vi "PRACTICA 1 REV.vi"() -> ()   [LabVIEW 2017]
panel:
  in  "stop":bool
  out "X+Y 2":dbl
  out "X+Y":dbl
  in  "Y":dbl
  in  "X":dbl
  out "C":dbl
  in  "B":dbl
  in  "A":dbl
  out "Boolean":bool
  # "-"
  # "="
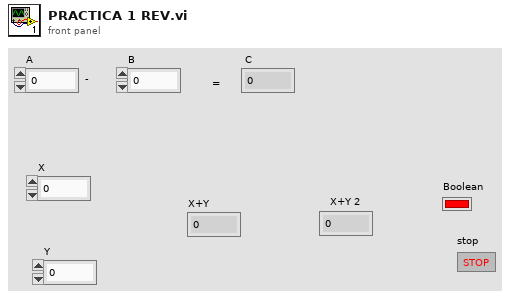
[diagram p1: front panel]
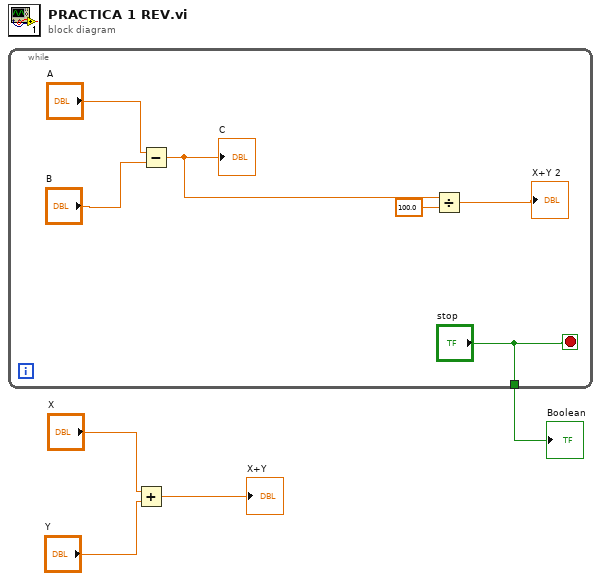
[diagram p0: block diagram]
diagram:
  n1 = while {
    tunnel: ["stop"] -> w1
    stop <- "stop" stop-if-true
    n2 = Subtract(x="A", y="B") -> (x-y=w7:dbl)
    "C" <- w7
    n3 = Divide(x=w7, y=100.0) -> (x/y=→"X+Y 2":dbl)
  }
  "Boolean" <- w1
  n4 = Add(x="X", y="Y") -> (x+y=→"X+Y":dbl)
